vi "set up new template project.vi"(8 "error in":errorcluster, 10 "project directory":path, 11 "VI path":path) -> (0 "error out":errorcluster, 3 "new project":path)   [LabVIEW 2014, in "CD model script.lvlib"]
uses:
  CD model script.lvlib
  CD Wizard - Execution Mode.ctl
  <vilib>/Utility/EditLVProj/Edit LVProj.lvlib
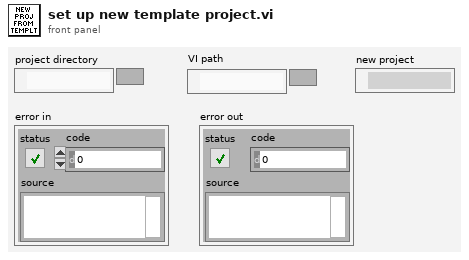
[diagram p1: front panel]
types:
  T1 = typedef "CD model script.lvlib/CD Wizard - Execution Mode.ctl" = enum16{"Asynchronous", "Inline HW Interface", "Inline Model Interface", "Inline Timing and Sync", "Asynchronous Timing and Sync"}
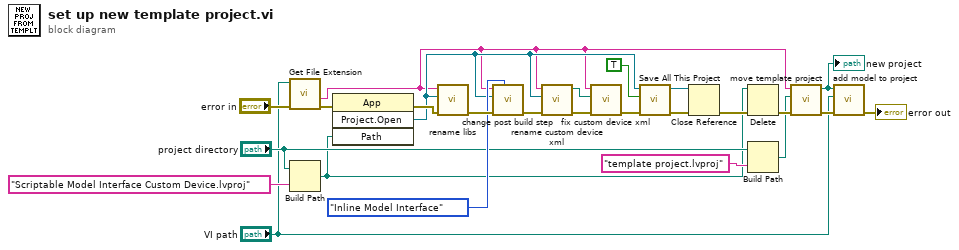
[diagram p0: block diagram]
diagram:
  n1 = call <vilib>:"Get File Extension.vi"("error in (no error)"="error in", "file"="VI path") -> ("error out"=w23:errorcluster, "filename without extension"=w10:string)  [unwired: 6 in, 2 out]
  n2 = Build Path(base path="project directory", name or relative path="Scriptable Model Interface Custom Device.lvproj") -> (appended path=w6:path)
  n3 = invoke class="App" method="Project.Open"(error in=w23, "Path"=w6) -> (error out=w22:errorcluster, "Project:Open"=w15:refnum<vi>)  [unwired: 2 in, 2 out]
  n4 = call "rename libs.vi"("error in (no error)"=w22, "User Project"=w15, "CD name"=w10) -> ("error out"=w21:errorcluster)  [unwired: 8 in]
  n5 = call "change post build step.vi"("CD Execution Mode"=CD_Wizard_-_Execution_Mode."Inline Model Interface", "error in (no error)"=w21, "User Project"=w15, "CD Name"=w10) -> ("error out"=w19:errorcluster)  [unwired: 7 in]
  n6 = call "rename custom device xml.vi"("error in"=w19, "User Project"=w15, "CD name"=w10) -> ("error out"=w18:errorcluster, "new xml path"=w17:path)  [unwired: 7 in]
  n7 = call "fix custom device xml.vi"("error in (no error)"=w18, "new xml path"=w17, "CD name"=w10) -> ("error out"=w16:errorcluster)  [unwired: 8 in]
  n8 = call <vilib>:"Save All This Project.vi"("error in (no error)"=w16, "Exclude Dependencies? (F)"=TRUE, "Project in"=w15) -> ("error out"=w13:errorcluster, "Project out"=w12:refnum<vi>)  [unwired: 7 in]
  n9 = Close Reference(reference=w12, error in (no error)=w13) -> (error out=w11:errorcluster)
  n10 = Delete(path (use dialog)=w6, error in=w11) -> (error out=w7:errorcluster)  [unwired: 3 in, 2 out]
  n11 = Build Path(base path="project directory", name or relative path="template project.lvproj") -> (appended path=w5:path)
  n12 = call "move template project.vi"("error in"=w7, "template path"=w5, "CD name"=w10) -> ("error out"=w4:errorcluster, "completed project"=w1:path)  [unwired: 7 in]
  "new project" <- w1
  n13 = call "add model to project.vi"("error in"=w4, "VI path"="VI path", "completed project"=w1) -> ("error out"=→"error out":errorcluster)  [unwired: 8 in]
